vi "Return Transfer Group.vi"(8 "error in (no error)":errorcluster, 10 "Transfer Group in":refnum<class "Transfer Group.lvclass">, 11 "Transceiver Thread in":refnum<class "Plugin Thread.lvclass">) -> (0 "error out":errorcluster, 2 "Transfer Group out":refnum<class "Transfer Group.lvclass">, 3 "Transceiver Thread out":refnum<class "Plugin Thread.lvclass">)   [LabVIEW 2017, in "DSF Core.lvlib" / "Plugin Thread.lvclass"]
uses:
  Thread/Plugin/Plugin Thread.lvclass
  Transfer Group/Transfer Group.lvclass
  Transfer Group/Transfer Group.lvclass/Transfer Group.ctl
  Timing/Timing.lvclass/Timing.ctl
  Transfer Group/Get Timing.vi
  Timing/Get Iteration.vi
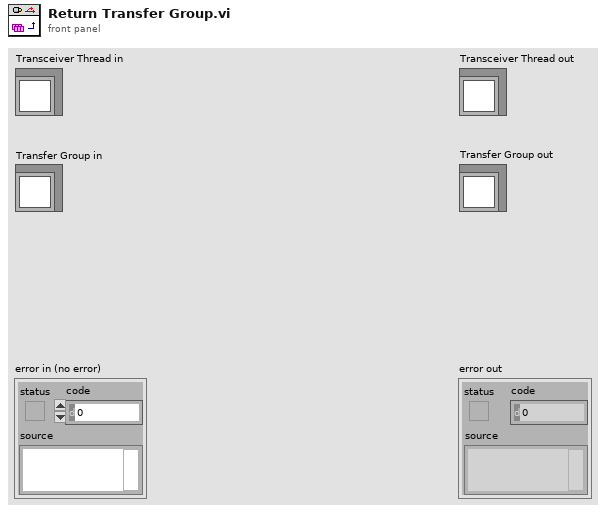
[diagram p1: front panel]
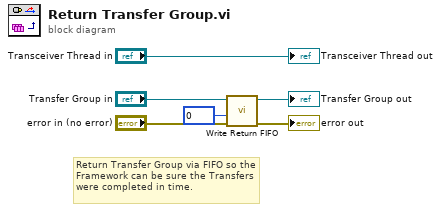
[diagram p0: block diagram]
diagram:
  # "Return Transfer Group via FIFO so the Framework can be sure the Transfers were completed in time."
  n1 = call "Write Return FIFO.vi"("error in (no error)"="error in (no error)", "timeout in ms (0)"=0, "Transfer Group in"="Transfer Group in") -> ("error out"=→"error out":errorcluster, "Transfer Group out"=→"Transfer Group out":refnum<class "Transfer Group.lvclass">)  [unwired: 6 in, 1 out]
  "Transceiver Thread out" <- "Transceiver Thread in"
